vi "monitor_pockel.vi"() -> ()   [LabVIEW 2009]
uses:
  <vilib>/DAQmx/configure/timing.llb/DAQmx Timing (Sample Clock).vi
  <vilib>/DAQmx/create/channels.llb/DAQmx Create Channel (AI-Voltage-Basic).vi
  <vilib>/Utility/file.llb/Write To Spreadsheet File (DBL).vi
  <vilib>/DAQmx/read.llb/DAQmx Read (Analog 2D DBL NChan NSamp).vi
  <vilib>/Analysis/NI_AALBase.lvlib
panel:
  in  "milliseconds to wait":u32=1000
  out "Waiting":bool
  out "Start time":timestamp
  out "Run time (s)":dbl format="%#_2g"
  in  "name or relative path":string="pockel_data.txt"
  out "Ratio":dbl
  in  "base path":path
  out "Chart":dbl(graph)
  out "Detector 2":dbl format="%0.2f"
  out "Detector 1":dbl format="%0.2f"
  in  "stop":bool
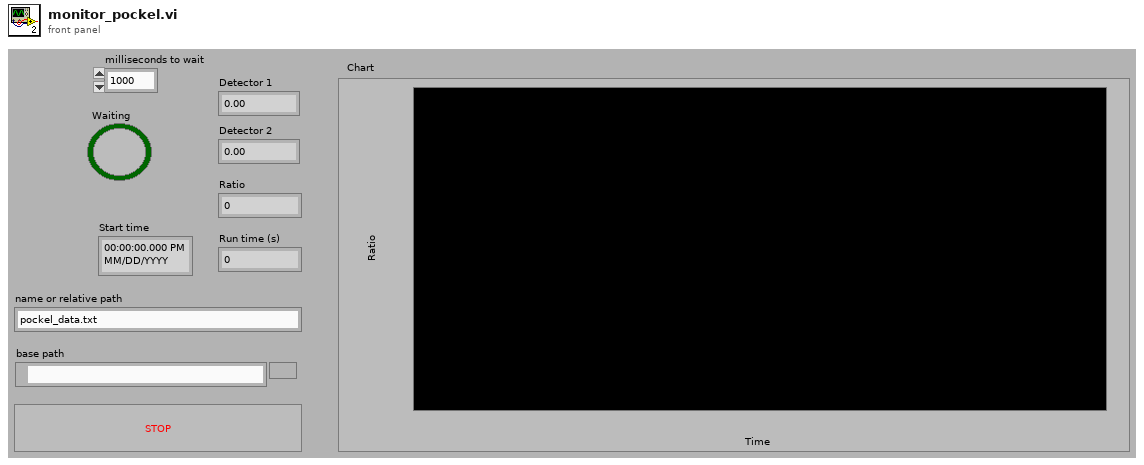
[diagram p1: front panel]
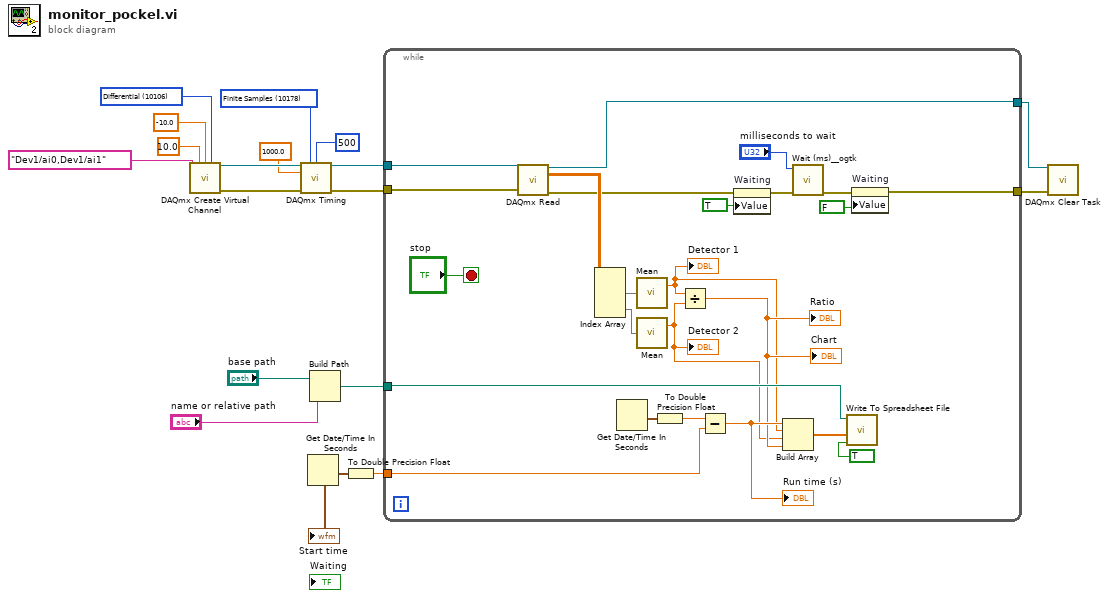
[diagram p0: block diagram]
diagram:
  w6 = 10178 items=["Finite Samples"=10178, "Continuous Samples"=10123, "Hardware Timed Single Point"=12522] ("sample mode")
  w16 = 10106 items=["default"=-1, "RSE"=10083, "NRSE"=10078, "Differential"=10106, "Pseudodifferential"=12529] ("input terminal configuration")
  n1 = call-poly <vilib>:"DAQmx Create Virtual Channel.vi"("maximum value"=10.0, "minimum value"=-10.0, "input terminal configuration"=w16, "physical channels"=tag "Dev1/ai0,Dev1/ai1") -> ("task out"=w11:refnum<k21>, "error out"=w9:errorcluster)  [unwired: 10 in]
  n2 = call-poly <vilib>:"DAQmx Timing.vi"("task/channels in"=w11, "sample mode"=w6, "samples per channel"=500, "rate"=1000.0, "error in"=w9) -> ("task out"=w10:refnum<k21>, "error out"=w8:errorcluster)  [unwired: 9 in]
  n3 = Get Date/Time In Seconds() -> (seconds since 1Jan1904=w4:timestamp)
  "Start time" <- w4
  n4 = Build Path(base path="base path", name or relative path="name or relative path") -> (appended path=w12:path)
  n5 = To Double Precision Float(number=w4) -> (double precision float=w3:dbl)
  n6 = while {
    tunnel: w10 -> [w42]
    tunnel: w8 -> [w40]
    tunnel: w12 -> [w38]
    tunnel: w3 -> [w30]
    tunnel: [w20] -> w2
    tunnel: [w19] -> w1
    stop <- "stop" stop-if-true
    n7 = call-poly <vilib>:"DAQmx Read.vi"("task/channels in"=w42, "error in"=w40) -> ("task out"=w19:refnum<k21>, "data"=w39:dbl[][], "error out"=w23:errorcluster)  [unwired: 11 in]
    n8 = Index Array(array=w39) -> (element #1=w34:dbl[], element #2=w33:dbl[])  [unwired: 4 in]
    n9 = Get Date/Time In Seconds() -> (seconds since 1Jan1904=w36:timestamp)
    n10 = call <vilib>:"Mean.vi"("X"=w34) -> ("mean"=w28:dbl)  [unwired: 1 out]
    "Detector 1" <- w28
    n11 = call <vilib>:"Mean.vi"("X"=w33) -> ("mean"=w27:dbl)  [unwired: 1 out]
    "Detector 2" <- w27
    n12 = To Double Precision Float(number=w36) -> (double precision float=w32:dbl)
    n13 = Divide(x=w28, y=w27) -> (x/y=w29:dbl)
    "Chart" <- w29
    "Ratio" <- w29
    n14 = Subtract(x=w32, y=w30) -> (x-y=w31:dbl)
    "Run time (s)" <- w31
    n15 = property on="Waiting" class="Bool (strict)"(error in=w23, "Value"=TRUE ("Waiting")) -> (error out=w22:errorcluster)  [unwired: 1 in, 1 out]
    n16 = Build Array(w31, w28, w27, w29) -> (w35:dbl[])
    n17 = call <userlib>:"Wait (ms)__ogtk.vi"("error in (no error)"=w22, "milliseconds to wait"="milliseconds to wait") -> ("error out"=w21:errorcluster)  [unwired: 8 in, 1 out]
    n18 = call-poly <vilib>:"Write To Spreadsheet File.vi"("append to file? (new file:F)"=TRUE, "1D data"=w35, "file path (dialog if empty)"=w38) -> ()  [unwired: 5 in, 1 out]
    n19 = property on="Waiting" class="Bool (strict)"(error in=w21, "Value"=FALSE ("Waiting")) -> (error out=w20:errorcluster)  [unwired: 1 in, 1 out]
  }
  n20 = call <vilib>:"DAQmx Clear Task.vi"("task in"=w1, "error in"=w2) -> ()  [unwired: 13 in, 1 out]
